vi "mappingProgramPublish.vi"() -> ()   [LabVIEW 2023]
uses:
  <vilib>/Math Plots/3D Math Plots/3D Comet/3D Comet XCtrl/3D Comet.xctl
  Program Files/National Instruments/LabVIEW 2023/examples/Instrument IO/Serial/support/Serial - Settings.ctl
  <vilib>/Instr/_visa.llb/VISA Configure Serial Port (Instr).vi
  <vilib>/Utility/file.llb/Read Delimited Spreadsheet (DBL).vi
  <vilib>/Math Plots/3D Math Plots/3D Comet/3D Comet Datatype/Public/Plot Helper (Matrices).vi
  Program Files/National Instruments/LabVIEW 2023/instr.lib/Marlin Instrument Driver/Marlin Instrument Driver.lvlib
  <vilib>/Math Plots/3D Math Plots/3D Comet/3D Comet Datatype/3D Comet Datatype.lvclass
panel:
  in  "Plot Path Button":bool
  out "MAPPING PATH VISUALIZER (mm)":refnum<class "3D Plot Datatype.lvclass">[](xcontrol)
  in  "Data Save Location":path
  in  "Close Probe\nClose 2":bool
  in  "Probe COM port":refnum<visa-resource-name>
  in  "Path":path caption="Pathing File Location"
  in  "Run Scan":bool
  in  "Custom Command":string
  out "Z":string
  out "Y":string
  out "X":string
  in  "Exit Scan\nClose":bool caption="Close\nClose"
  out "Initialized":bool
  in  "Initialize":bool
  in  "COM port":refnum<visa-resource-name> caption="Printer Chassis COM port"
  in  "Speed":u32=1000 caption="mm/min"
  in  "Distance":dbl=2.0 caption="mm"
  in  "Home all":bool caption="ALL"
  in  "Home Z":bool
  in  "Z-":bool
  in  "Z+":bool
  in  "Home XY":bool
  in  "XY-":bool
  in  "X-":bool
  in  "XY+":bool
  in  "X-Y+":bool
  in  "Y-":bool
  in  "X+Y-":bool
  in  "X+":bool
  in  "Y+":bool
  # "ENSURE DATA SAVING LOCATION, PATHING FILE LOCATION, AND COM PORTS ARE SELECTED, \nAND PRINTER CHASSIS IS INITALIZED BEFORE ATTEMPTING TO RUN SCAN."
  # "CAUTION: Z-AXIS MOVEMENT MAY CRASH SENSOR INTO PRINT BED."
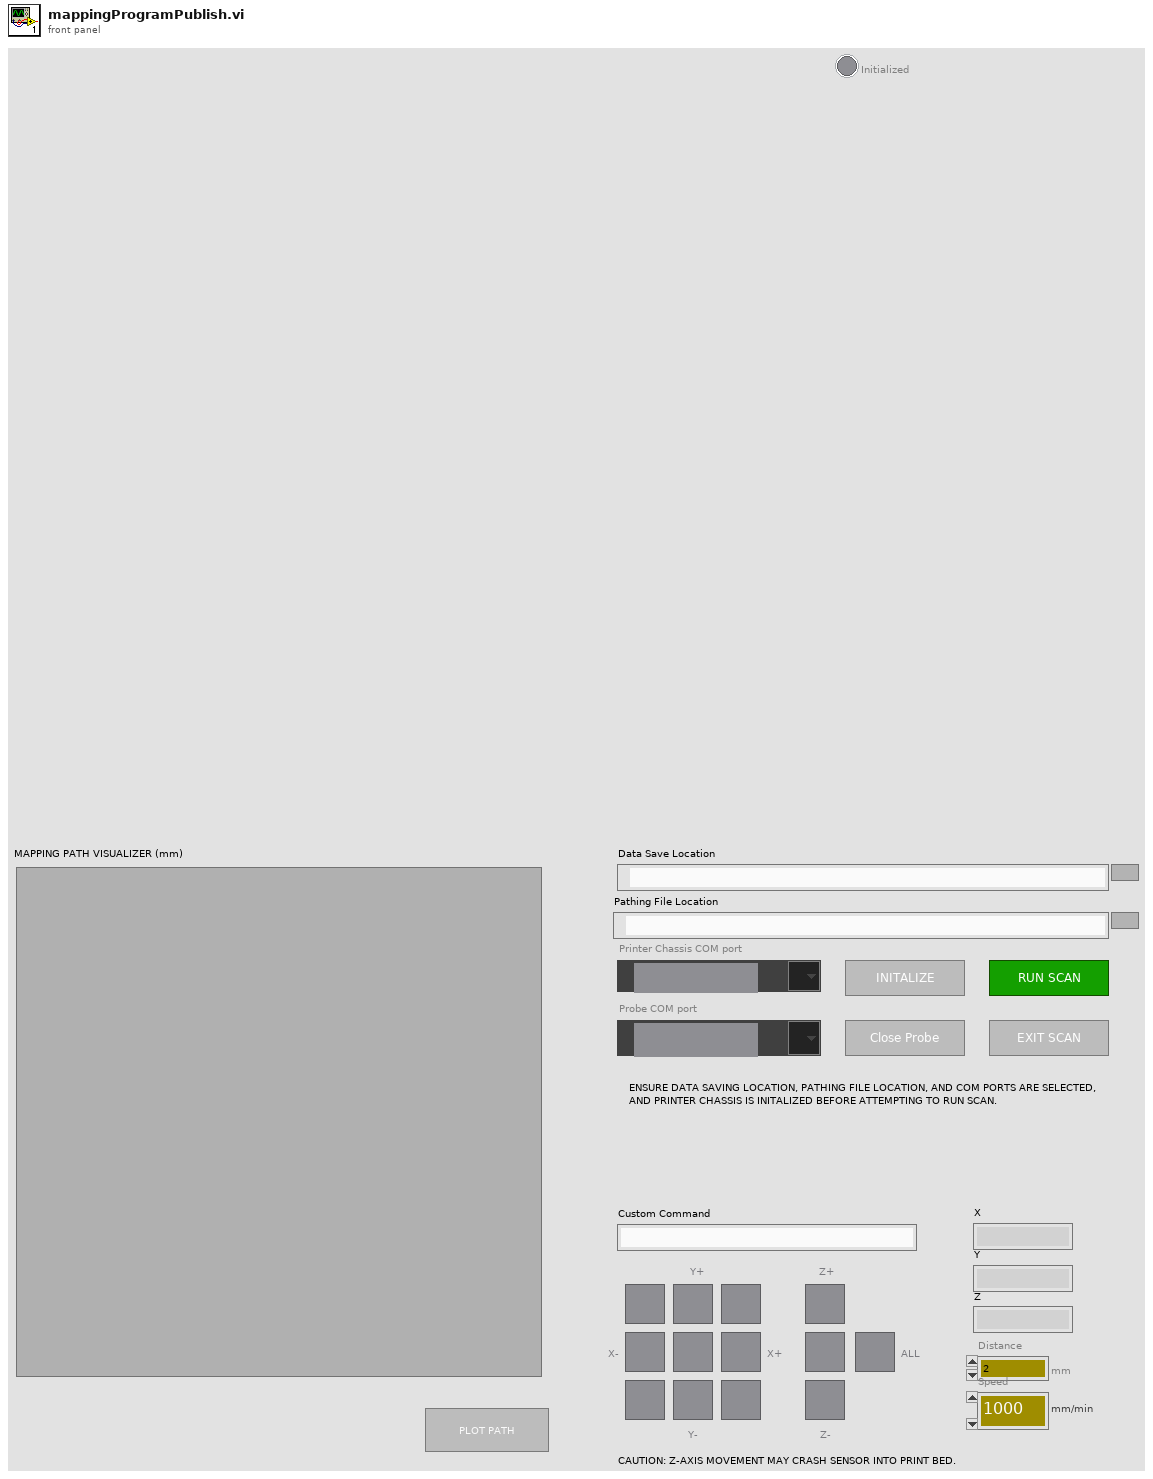
[diagram p1: front panel]
types:
  T1 = enum16{"open", "replace", "create", "open or create", "replace or create", "replace or create with confirmation"}
  T2 = typedef "Serial - Settings.ctl" = cluster{"baud rate":u32, "data bits":u16, "parity":enum16{"None", "Odd", "Even", "Mark", "Space"}, "stop bits":u16, "flow control":u16}
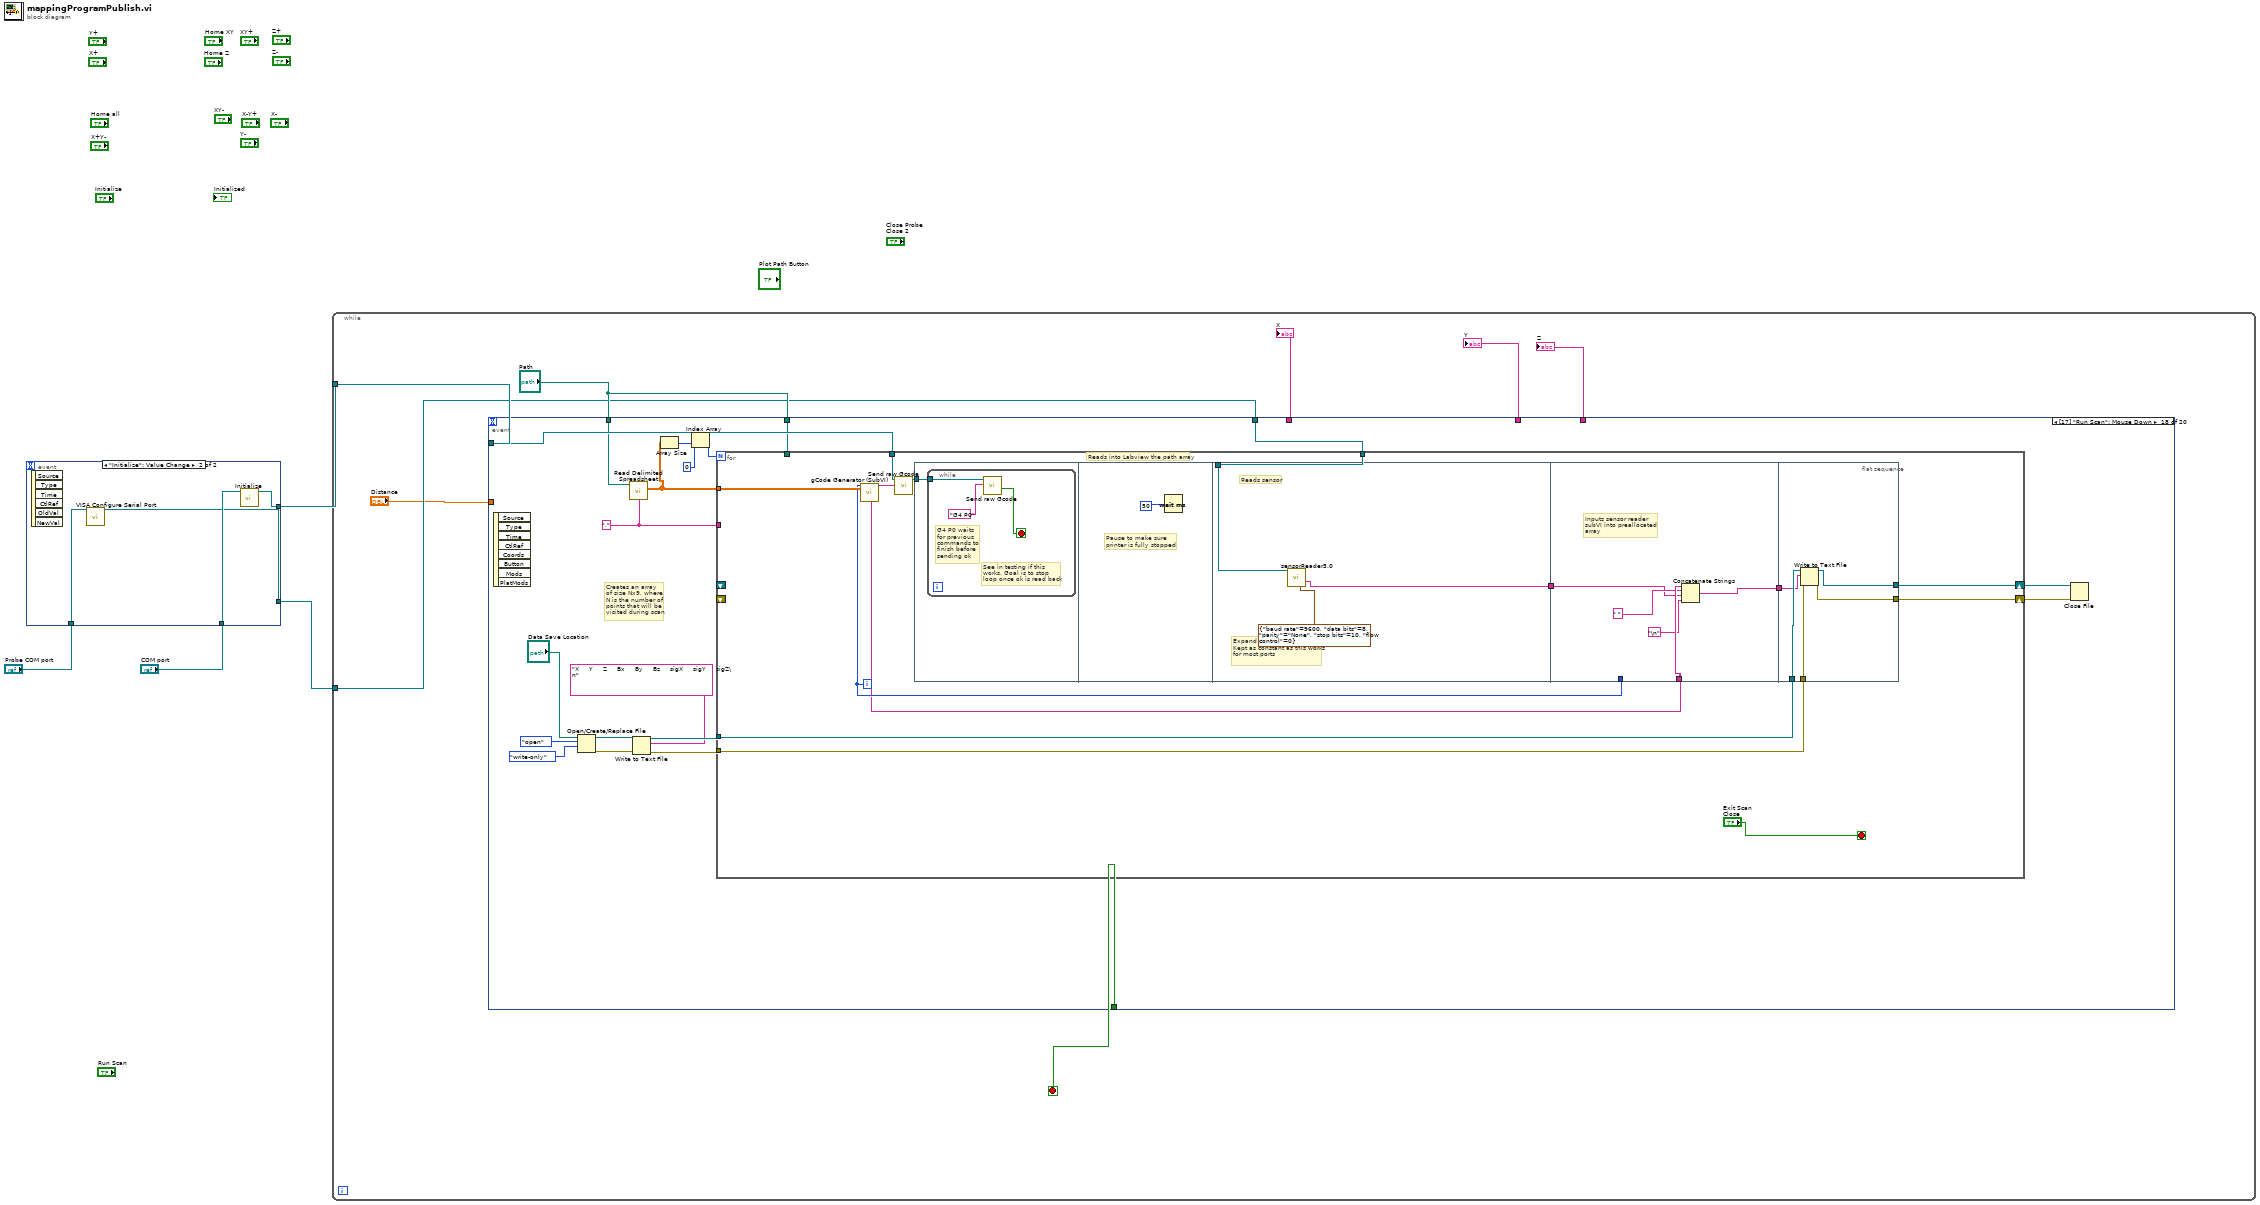
[diagram p0: block diagram]
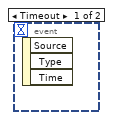
[diagram p2: hidden frame]
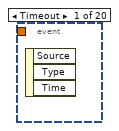
[diagram p3: hidden frame]
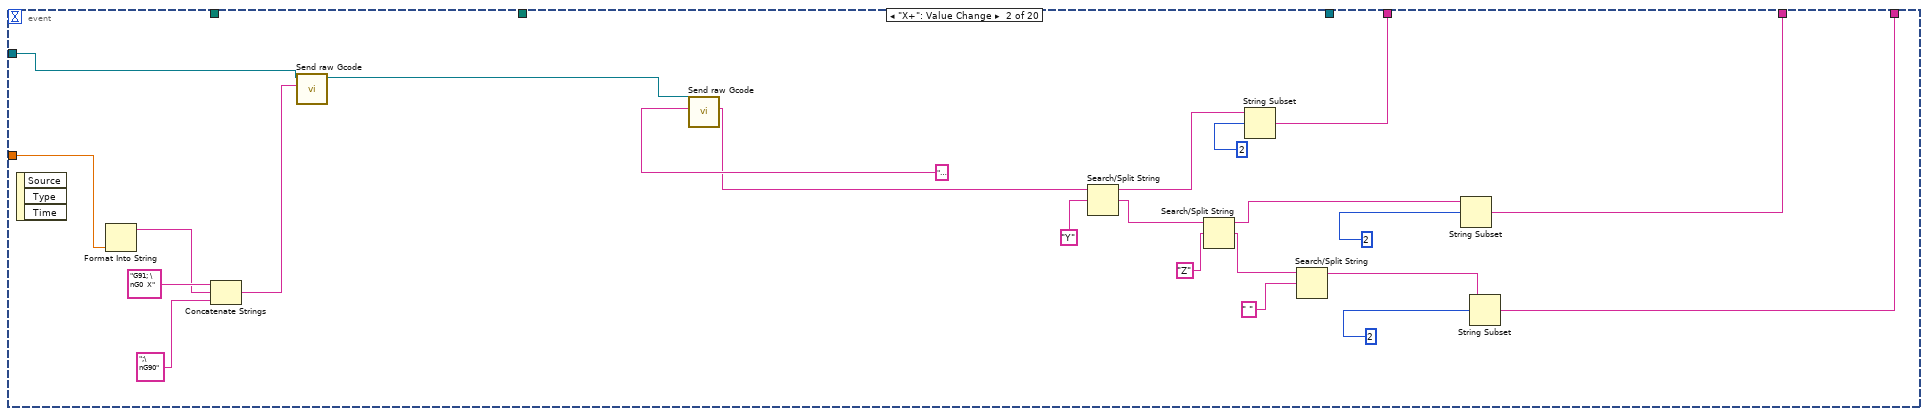
[diagram p4: hidden frame]
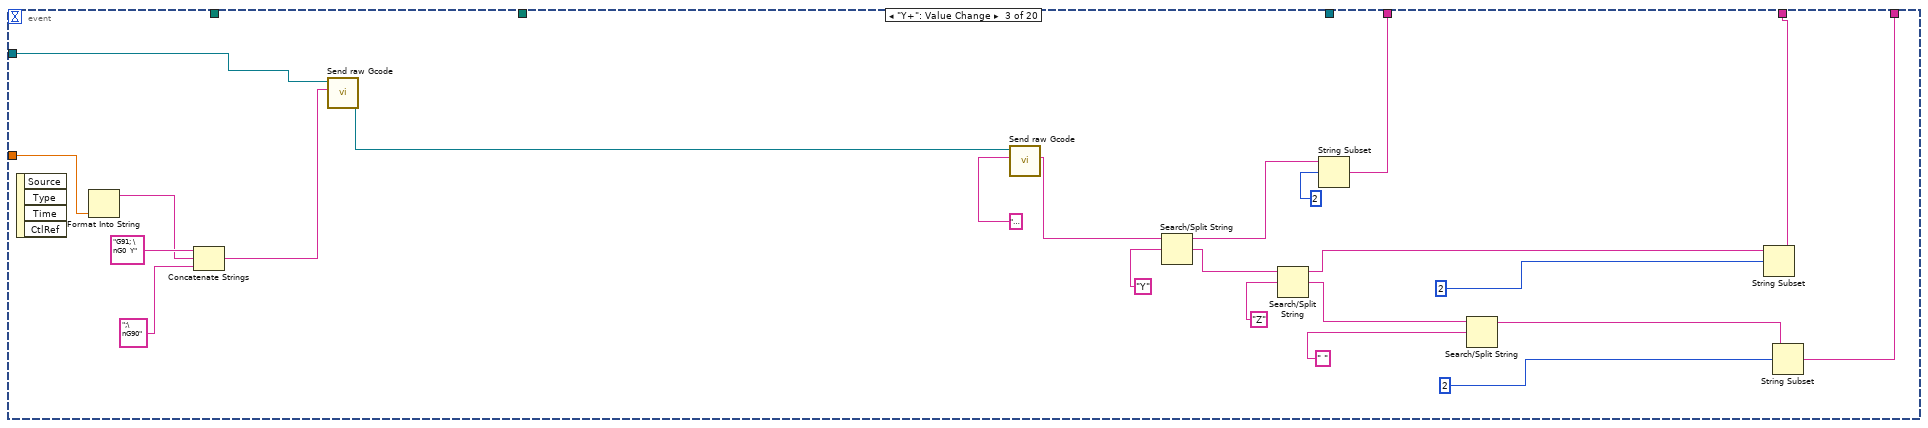
[diagram p5: hidden frame]
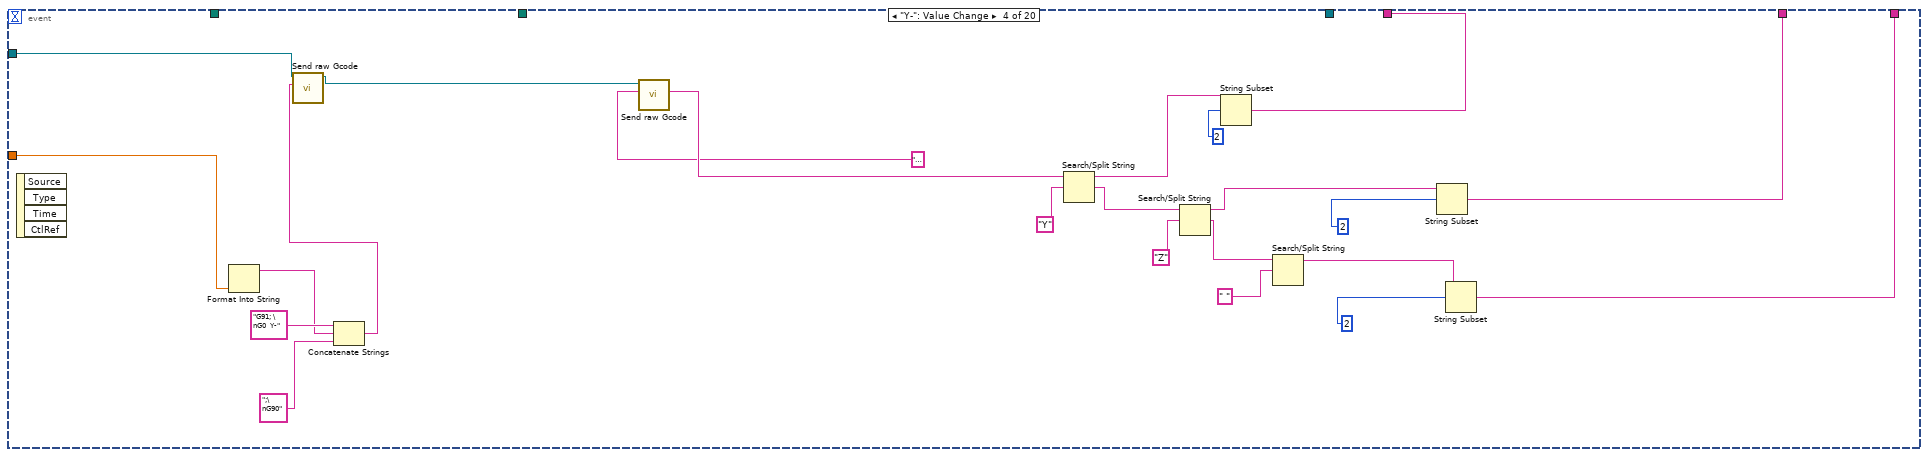
[diagram p6: hidden frame]
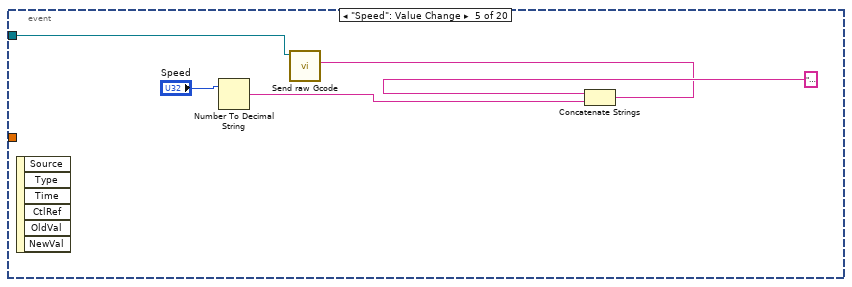
[diagram p7: hidden frame]
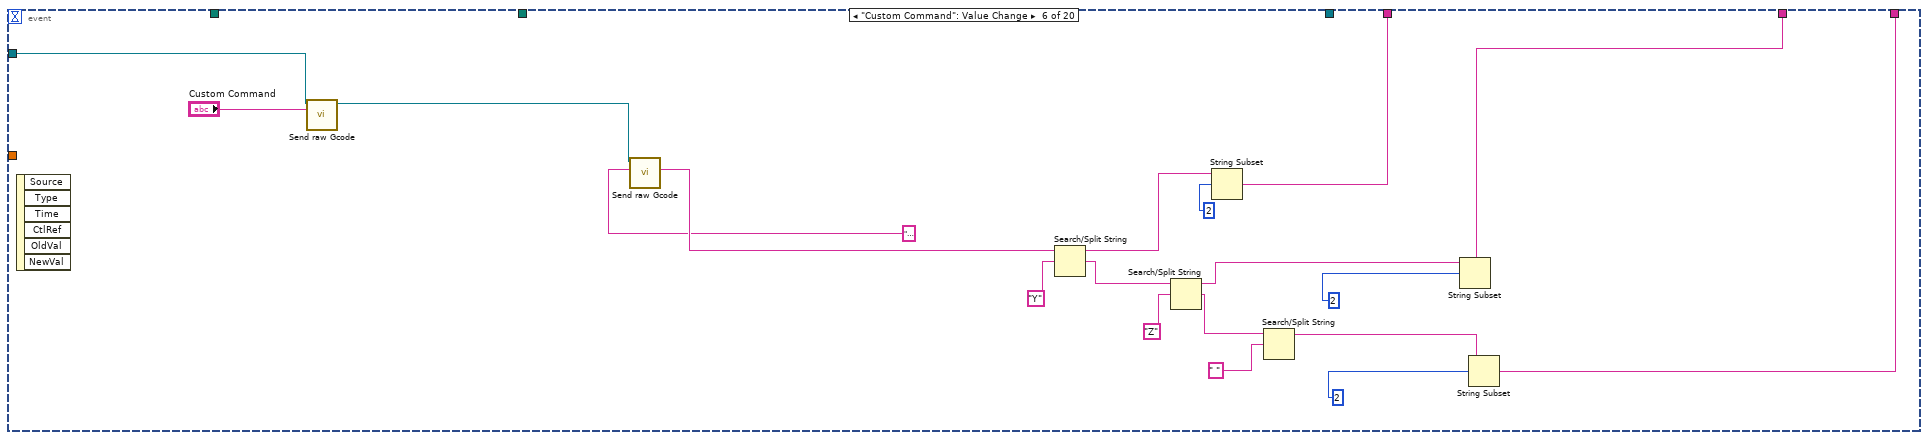
[diagram p8: hidden frame]
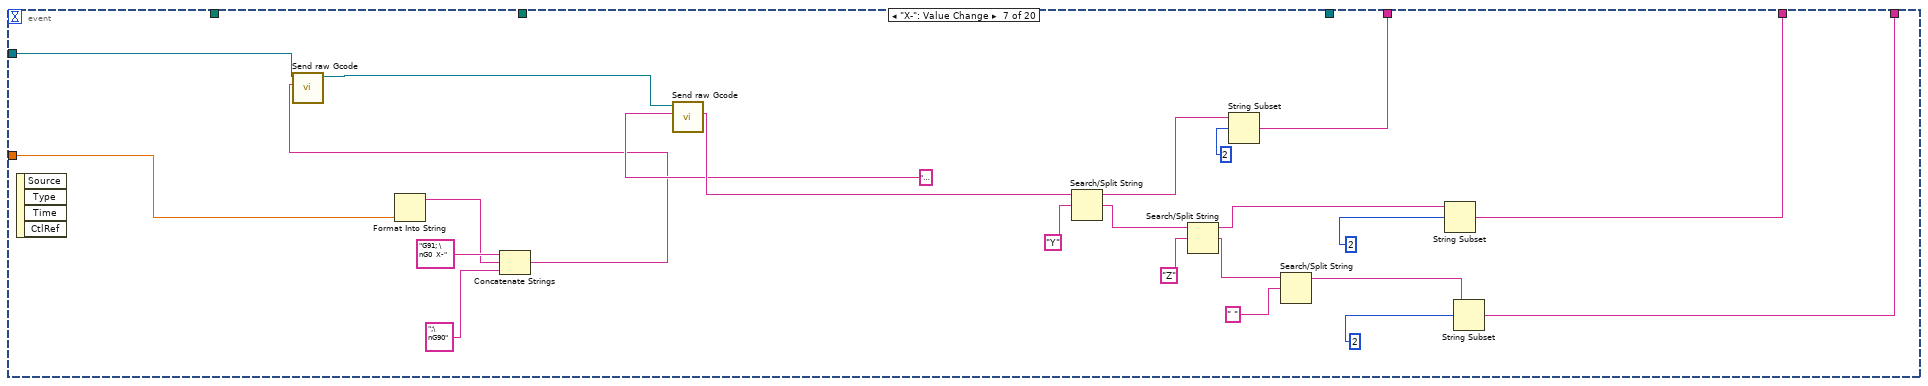
[diagram p9: hidden frame]
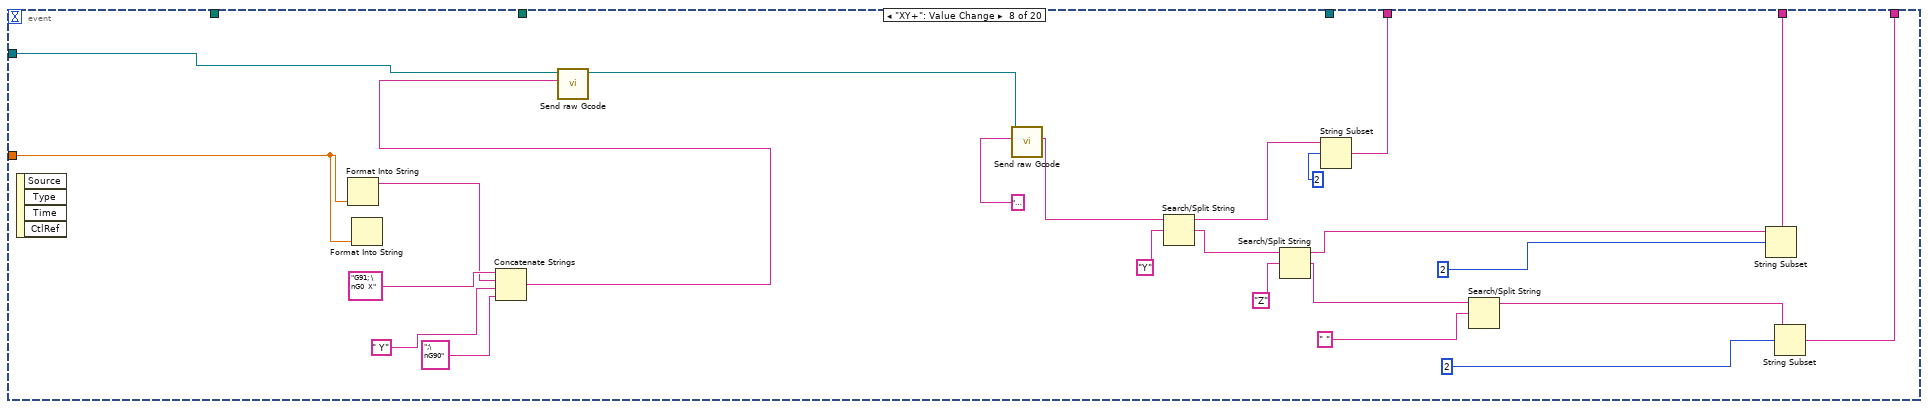
[diagram p10: hidden frame]
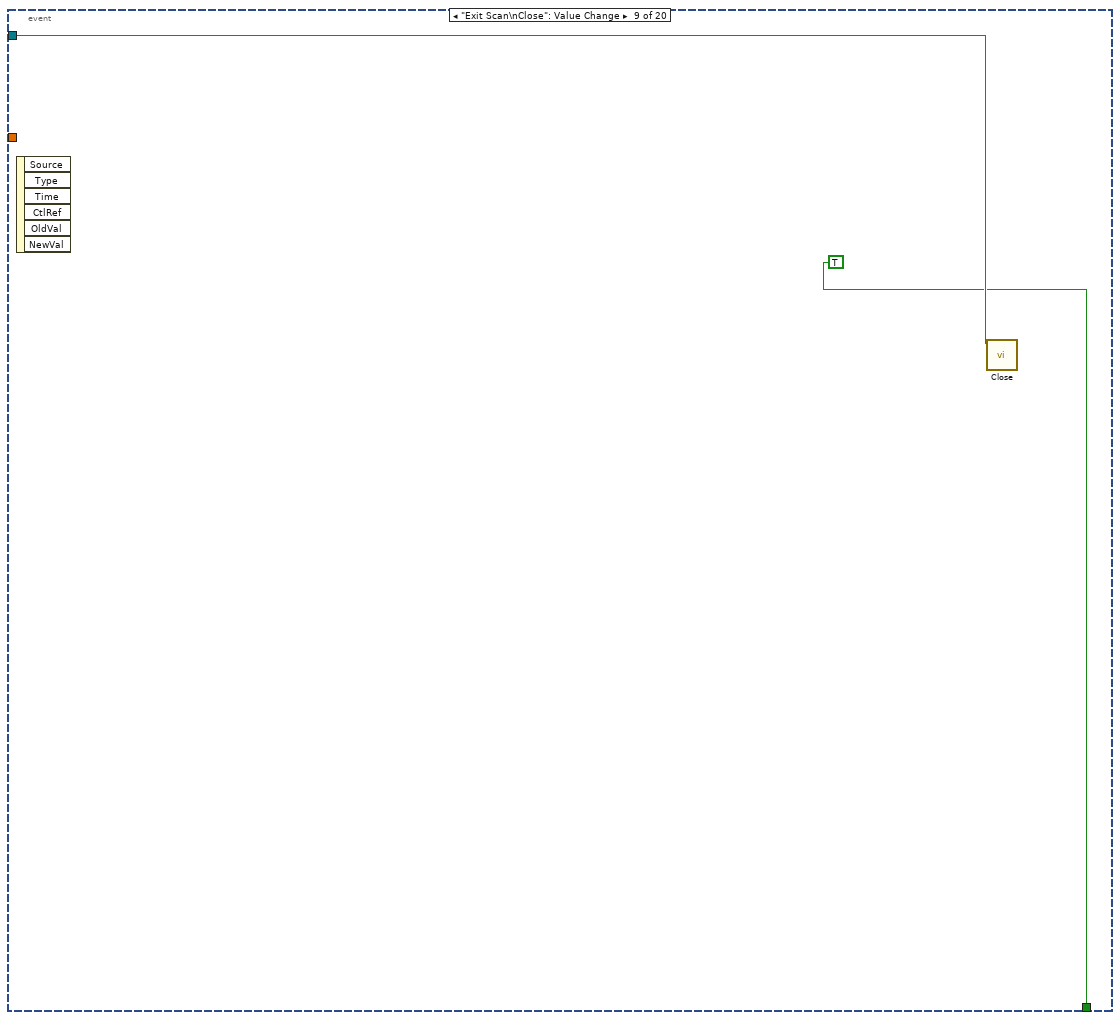
[diagram p11: hidden frame]
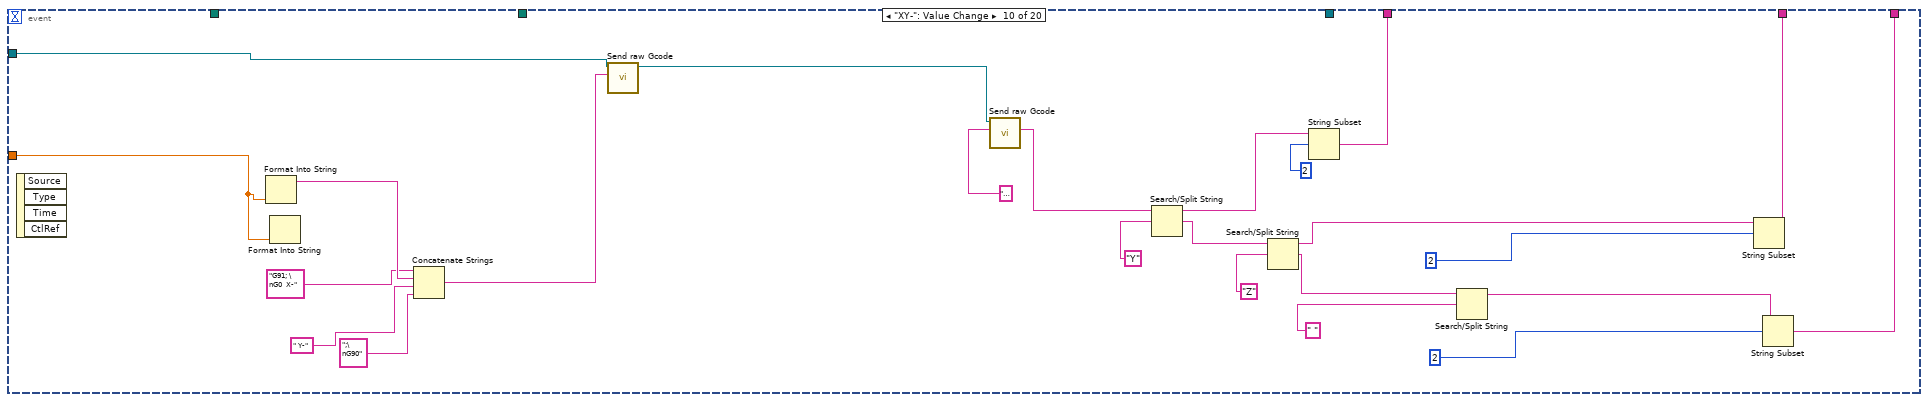
[diagram p12: hidden frame]
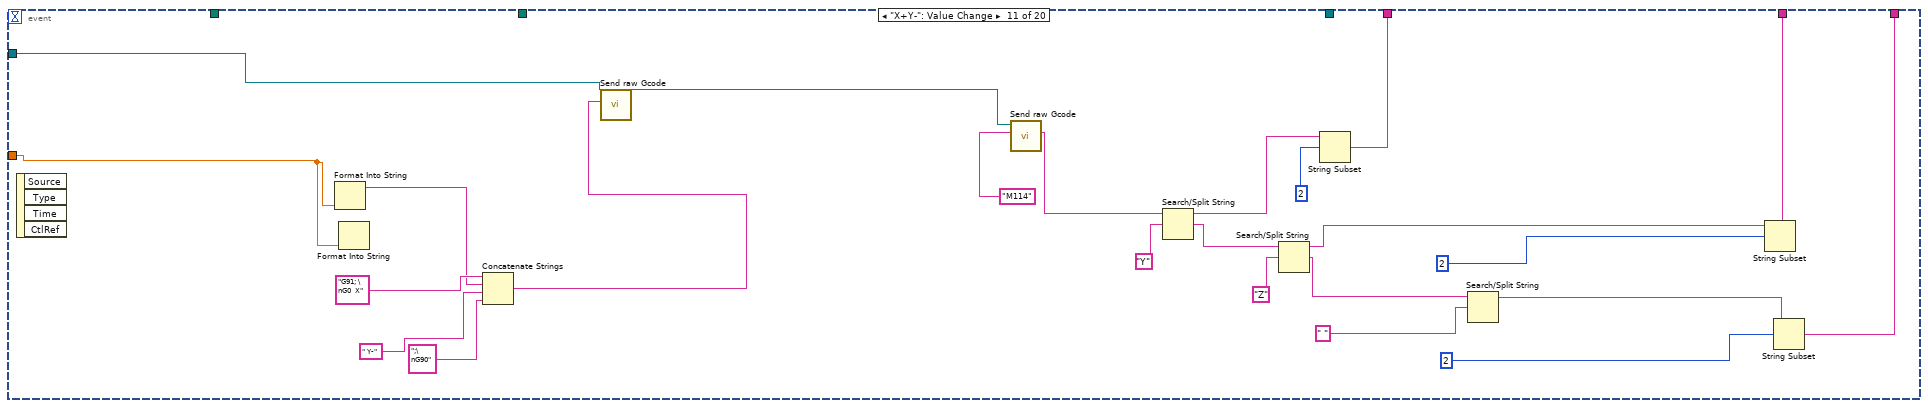
[diagram p13: hidden frame]
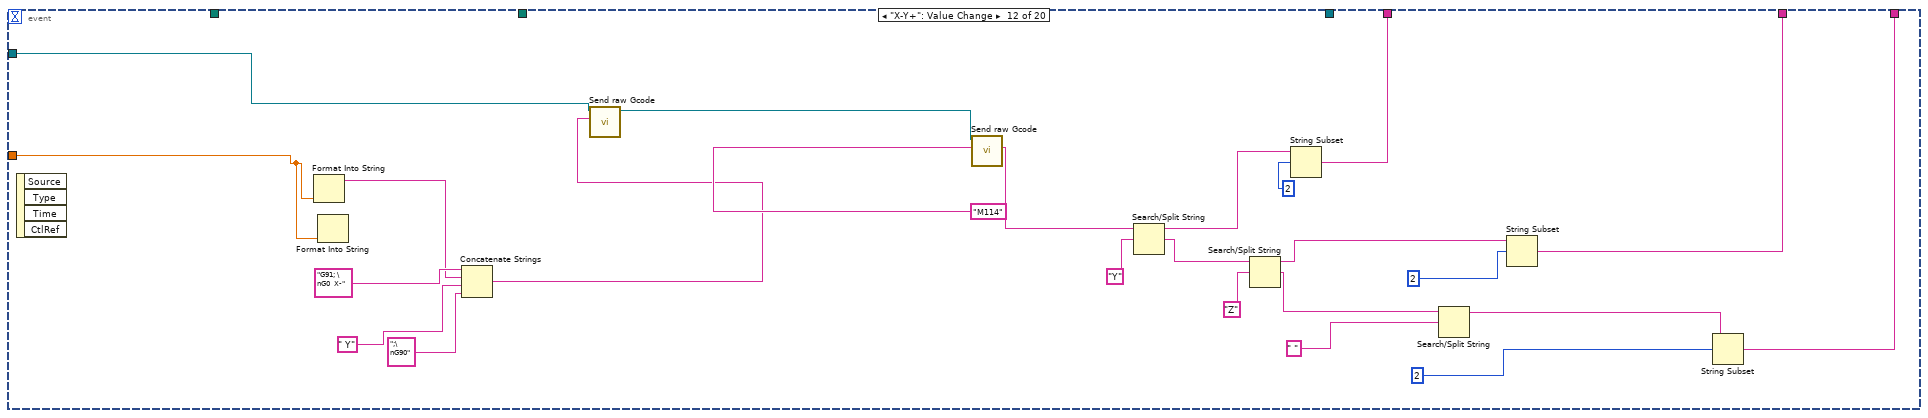
[diagram p14: hidden frame]
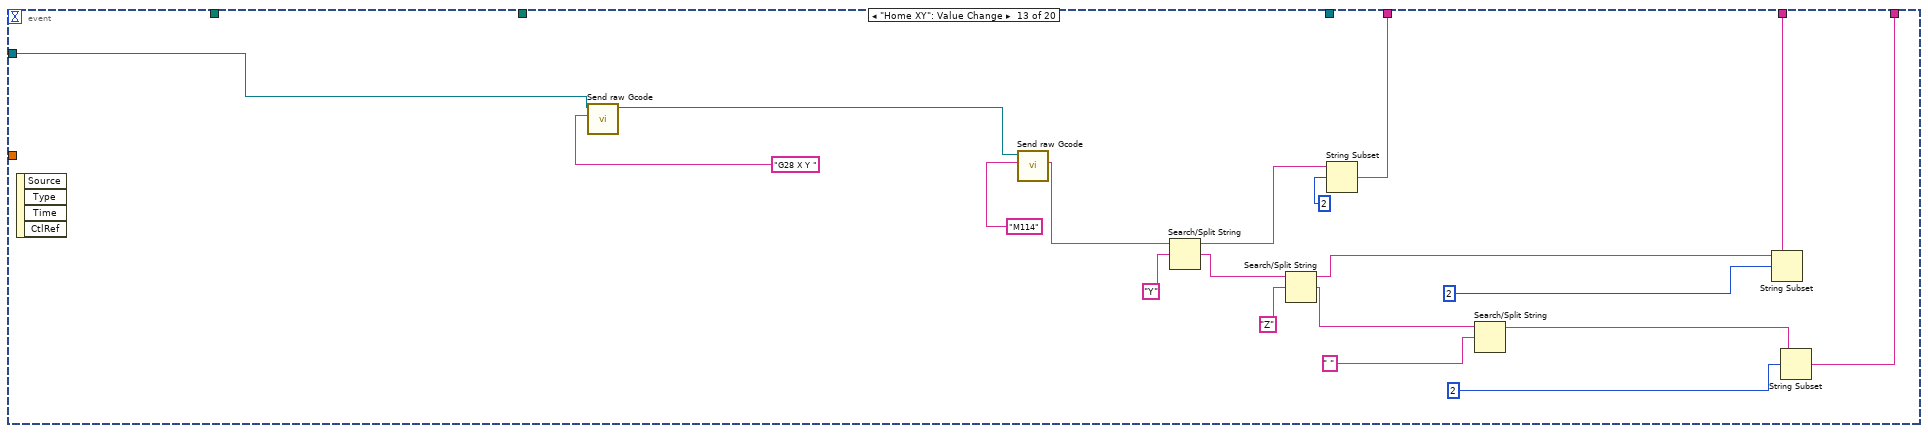
[diagram p15: hidden frame]
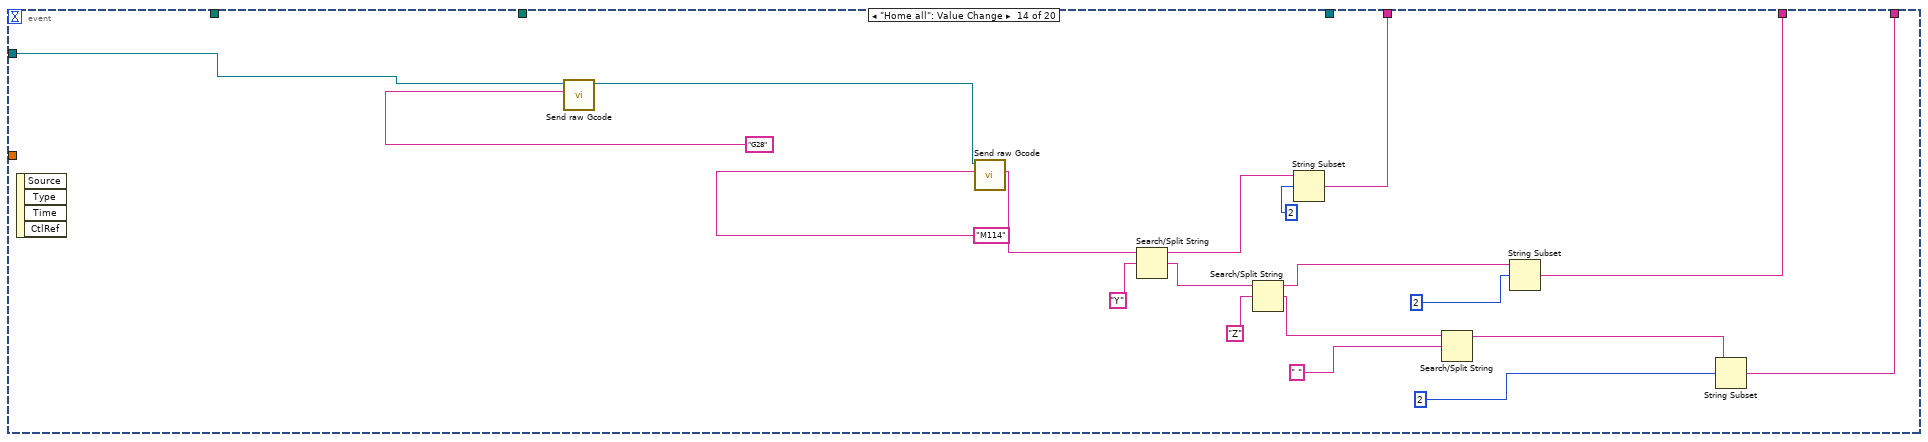
[diagram p16: hidden frame]
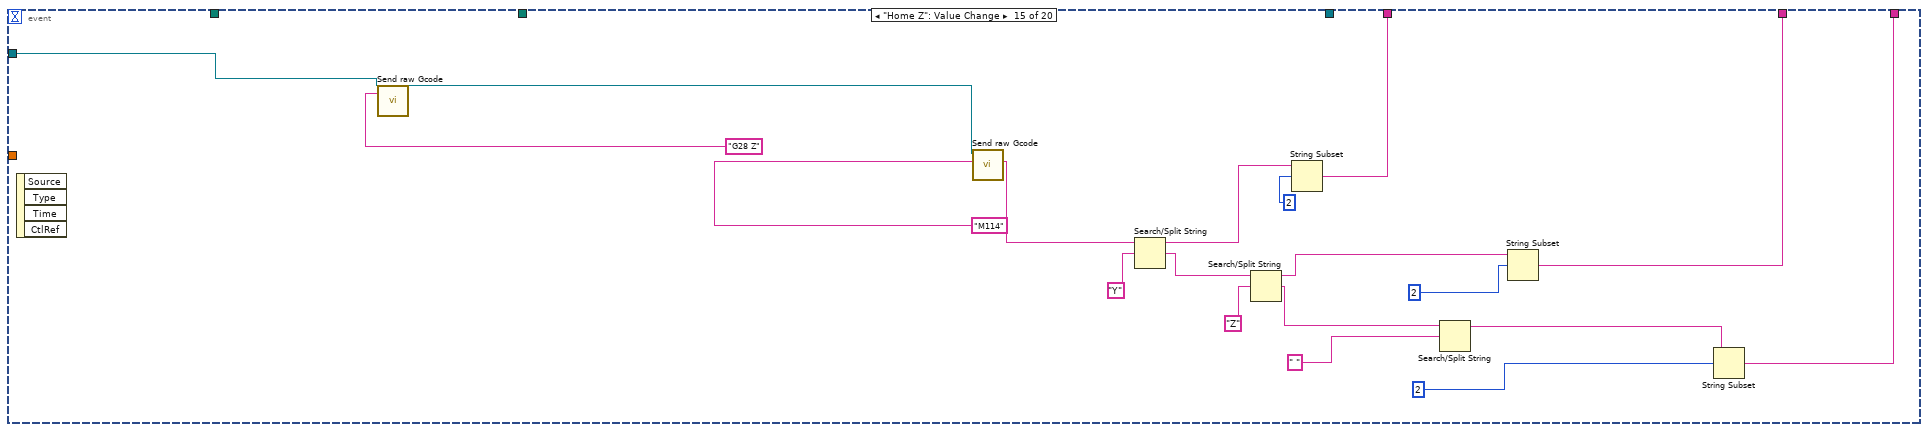
[diagram p17: hidden frame]
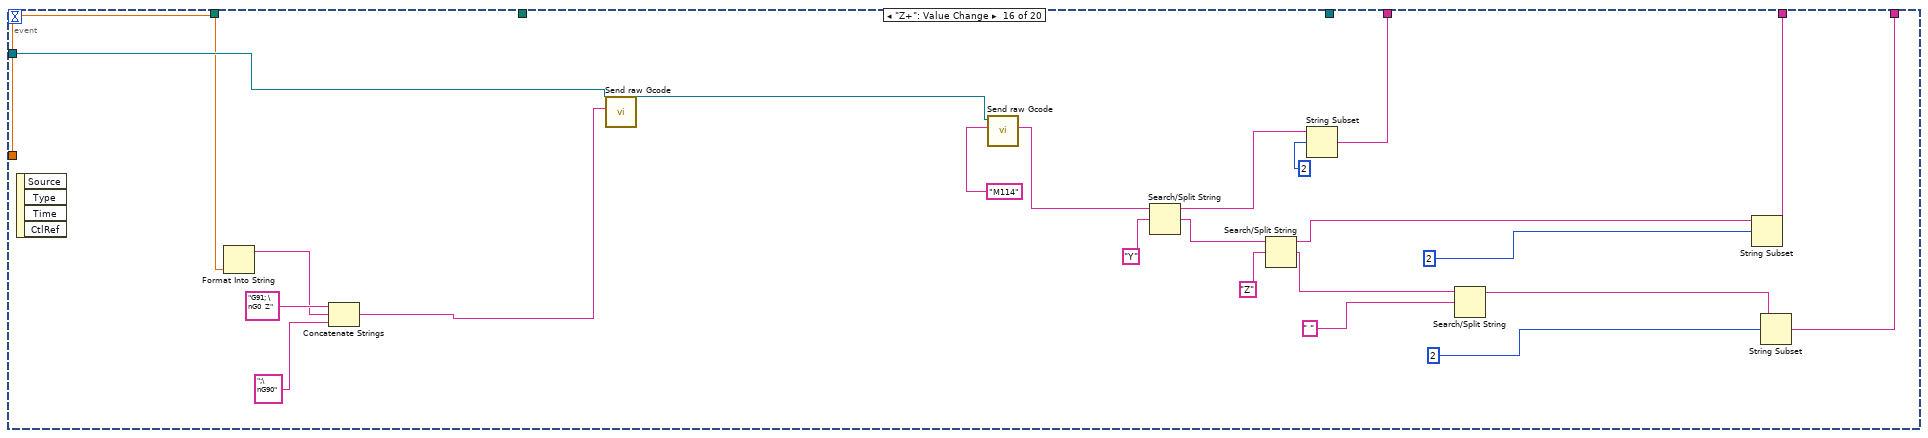
[diagram p18: hidden frame]
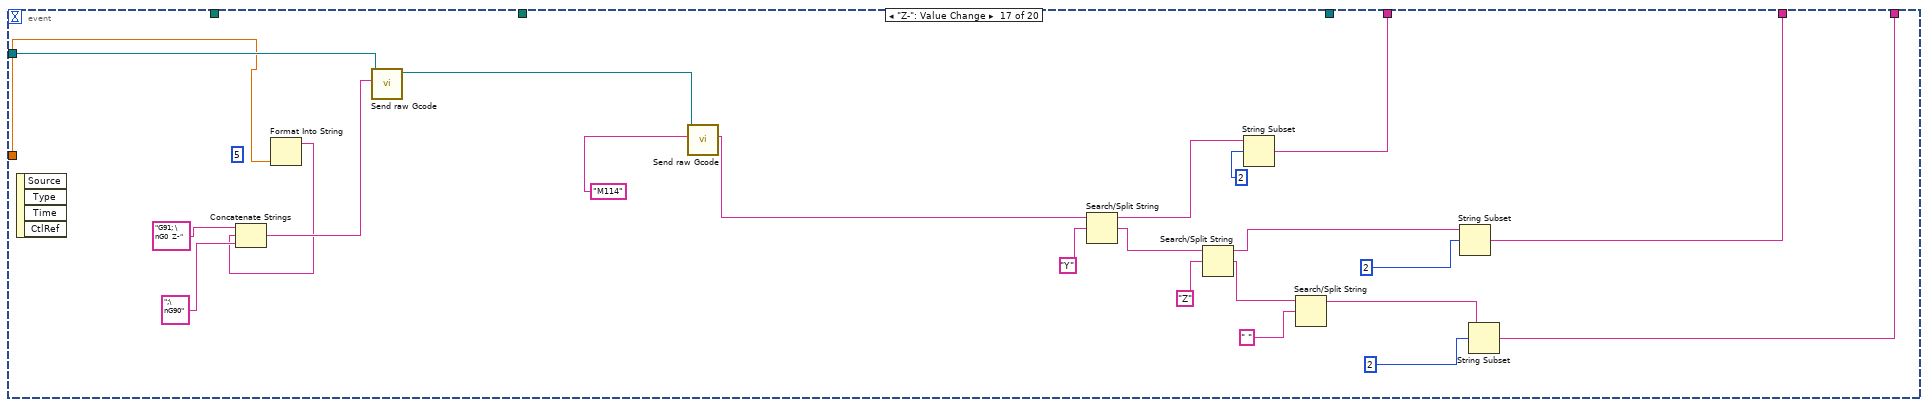
[diagram p19: hidden frame]
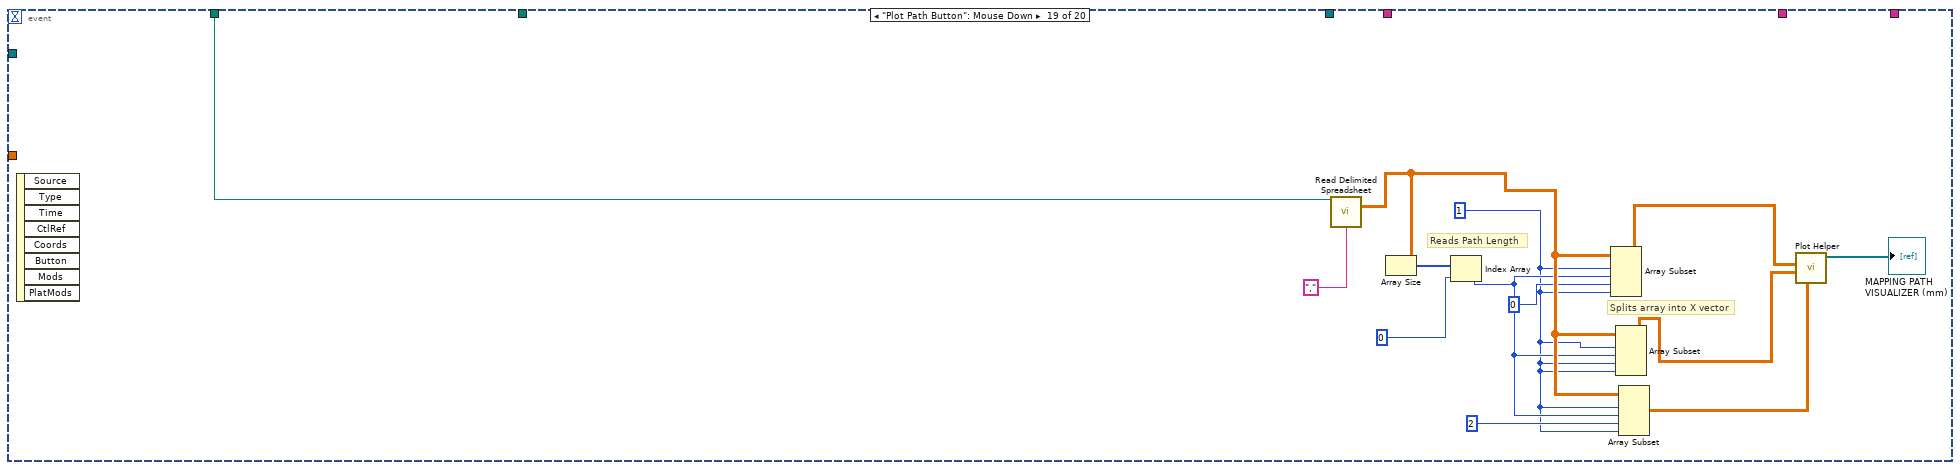
[diagram p20: hidden frame]
diagram:
  n1 = event shown="[1] \"Initialize\": Value Change" {
    selector: _ -> [_ _]
    dyn-events: _ -> [_ _]
    timeout: _ -> [_ _]
    tunnel: [_ w8] -> w3
    tunnel: "COM port" -> [_ w7]
    tunnel: "Probe COM port" -> [_ w6]
    tunnel: [_ w5] -> w1
    event Timeout {
      n2 = event-data() -> ()  [unwired: 1 in, 3 out]
    }
    event "Initialize": Value Change {
      n3 = event-data() -> ()  [unwired: 1 in, 6 out]
      n4 = call-poly "VISA Configure Serial Port"("VISA resource name"=w6) -> ("VISA resource name out"=w5:refnum<visa-resource-name>)  [unwired: 13 in, 1 out]
      n5 = call "Initialize.vi"("VISA resource name"=w7) -> ("VISA resource name out"=w8:refnum<visa-resource-name>)  [unwired: 9 in, 1 out]
    }
  }
  n6 = while {
    tunnel: w3 -> [w16]
    tunnel: w1 -> [w10]
    stop <- w15 stop-if-true
    n7 = event shown="[17] \"Run Scan\": Mouse Down" {
      selector: _ -> [_ _ _ _ _ _ _ _ _ _ _ _ _ _ _ _ _ _ _ _]
      dyn-events: _ -> [_ _ _ _ _ _ _ _ _ _ _ _ _ _ _ _ _ _ _ _]
      timeout: _ -> [_ _ _ _ _ _ _ _ _ _ _ _ _ _ _ _ _ _ _ _]
      tunnel: w16 -> [_ w38 w62 w85 w88 w109 w132 w156 w158 w182 w206 w230 w248 w267 w286 w310 w333 w351 _ _]
      tunnel: [_ _ _ _ _ _ _ _ TRUE _ _ _ _ _ _ _ _ _ _ _] -> w15
      tunnel: [_ w26 w47 w70 _ w94 w117 w141 _ w167 w191 w215 w233 w252 w271 w295 w318 _ _ _] -> w14
      tunnel: [_ w25 w46 w69 _ w93 w116 w140 _ w166 w190 w214 w232 w251 w270 w294 w317 _ _ _] -> w13
      tunnel: [_ w24 w45 w68 _ w92 w115 w139 _ w165 w189 w213 w231 w250 w269 w293 w316 _ _ _] -> w12
      tunnel: w10 -> [_ _ _ _ _ _ _ _ _ _ _ _ _ _ _ _ _ w348 _ w398]
      tunnel: "Path" -> [_ _ _ _ _ _ _ _ _ _ _ _ _ _ _ _ _ w346 w385 _]
      tunnel: "Path" -> [_ _ _ _ _ _ _ _ _ _ _ _ _ _ _ _ _ w345 _ _]
      tunnel: "Distance" -> [_ w17 w40 w63 _ _ w110 w137 _ w160 w184 w208 _ _ _ w289 w312 _ _ _]
      event Timeout {
        n8 = event-data() -> ()  [unwired: 1 in, 3 out]
      }
      event "X+": Value Change {
        n9 = event-data() -> ()  [unwired: 1 in, 3 out]
        n10 = Format Into String(w17) -> (resulting string=w19:string)  [unwired: 3 in, 1 out]
        n11 = Concatenate Strings("G91; \nG0  X", w19, ";\nG90") -> (w18:string)
        n12 = call "Send raw Gcode.vi"("Gcode"=w18, "VISA resource name"=w38) -> ("VISA resource name out"=w22:refnum<visa-resource-name>)  [unwired: 6 in, 3 out]
        n13 = call "Send raw Gcode.vi"("Gcode"="M114", "VISA resource name"=w22) -> ("read buffer"=w23:string)  [unwired: 6 in, 3 out]
        n14 = Search/Split String(string=w23, search string/char (-)="Y") -> (substring before match=w28:string, match + rest of string=w27:string)  [unwired: 1 in, 1 out]
        n15 = Search/Split String(string=w27, search string/char (-)="Z") -> (substring before match=w30:string, match + rest of string=w31:string)  [unwired: 1 in, 1 out]
        n16 = String Subset(string=w28, offset (0)=2) -> (substring=w26:string)  [unwired: 1 in]
        n17 = Search/Split String(string=w31, search string/char (-)=" ") -> (substring before match=w29:string)  [unwired: 1 in, 2 out]
        n18 = String Subset(string=w30, offset (0)=2) -> (substring=w25:string)  [unwired: 1 in]
        n19 = String Subset(string=w29, offset (0)=2) -> (substring=w24:string)  [unwired: 1 in]
      }
      event "Y+": Value Change {
        n20 = event-data() -> ()  [unwired: 1 in, 4 out]
        n21 = Format Into String(w40) -> (resulting string=w42:string)  [unwired: 3 in, 1 out]
        n22 = Concatenate Strings("G91; \nG0  Y", w42, ";\nG90") -> (w41:string)
        n23 = call "Send raw Gcode.vi"("Gcode"=w41, "VISA resource name"=w62) -> ("VISA resource name out"=w48:refnum<visa-resource-name>)  [unwired: 6 in, 3 out]
        n24 = call "Send raw Gcode.vi"("Gcode"="M114", "VISA resource name"=w48) -> ("read buffer"=w61:string)  [unwired: 6 in, 3 out]
        n25 = Search/Split String(string=w61, search string/char (-)="Y") -> (substring before match=w59:string, match + rest of string=w60:string)  [unwired: 1 in, 1 out]
        n26 = Search/Split String(string=w60, search string/char (-)="Z") -> (substring before match=w57:string, match + rest of string=w56:string)  [unwired: 1 in, 1 out]
        n27 = String Subset(string=w59, offset (0)=2) -> (substring=w47:string)  [unwired: 1 in]
        n28 = Search/Split String(string=w56, search string/char (-)=" ") -> (substring before match=w58:string)  [unwired: 1 in, 2 out]
        n29 = String Subset(string=w57, offset (0)=2) -> (substring=w46:string)  [unwired: 1 in]
        n30 = String Subset(string=w58, offset (0)=2) -> (substring=w45:string)  [unwired: 1 in]
      }
      event "Y-": Value Change {
        n31 = event-data() -> ()  [unwired: 1 in, 4 out]
        n32 = Format Into String(w63) -> (resulting string=w65:string)  [unwired: 3 in, 1 out]
        n33 = Concatenate Strings("G91; \nG0  Y-", w65, ";\nG90") -> (w64:string)
        n34 = call "Send raw Gcode.vi"("Gcode"=w64, "VISA resource name"=w85) -> ("VISA resource name out"=w71:refnum<visa-resource-name>)  [unwired: 6 in, 3 out]
        n35 = call "Send raw Gcode.vi"("Gcode"="M114", "VISA resource name"=w71) -> ("read buffer"=w79:string)  [unwired: 6 in, 3 out]
        n36 = Search/Split String(string=w79, search string/char (-)="Y") -> (substring before match=w81:string, match + rest of string=w80:string)  [unwired: 1 in, 1 out]
        n37 = Search/Split String(string=w80, search string/char (-)="Z") -> (substring before match=w83:string, match + rest of string=w84:string)  [unwired: 1 in, 1 out]
        n38 = String Subset(string=w81, offset (0)=2) -> (substring=w70:string)  [unwired: 1 in]
        n39 = Search/Split String(string=w84, search string/char (-)=" ") -> (substring before match=w82:string)  [unwired: 1 in, 2 out]
        n40 = String Subset(string=w83, offset (0)=2) -> (substring=w69:string)  [unwired: 1 in]
        n41 = String Subset(string=w82, offset (0)=2) -> (substring=w68:string)  [unwired: 1 in]
      }
      event "Speed": Value Change {
        n42 = event-data() -> ()  [unwired: 1 in, 6 out]
        n43 = Number To Decimal String(number="Speed") -> (decimal integer string=w89:string)  [unwired: 1 in]
        n44 = Concatenate Strings("G0 F", w89) -> (w86:string)
        n45 = call "Send raw Gcode.vi"("Gcode"=w86, "VISA resource name"=w88) -> ()  [unwired: 6 in, 4 out]
      }
      event "Custom Command": Value Change {
        n46 = event-data() -> ()  [unwired: 1 in, 6 out]
        n47 = call "Send raw Gcode.vi"("Gcode"="Custom Command", "VISA resource name"=w109) -> ("VISA resource name out"=w91:refnum<visa-resource-name>)  [unwired: 6 in, 3 out]
        n48 = call "Send raw Gcode.vi"("Gcode"="M114", "VISA resource name"=w91) -> ("read buffer"=w102:string)  [unwired: 6 in, 3 out]
        n49 = Search/Split String(string=w102, search string/char (-)="Y") -> (substring before match=w104:string, match + rest of string=w103:string)  [unwired: 1 in, 1 out]
        n50 = Search/Split String(string=w103, search string/char (-)="Z") -> (substring before match=w106:string, match + rest of string=w107:string)  [unwired: 1 in, 1 out]
        n51 = String Subset(string=w104, offset (0)=2) -> (substring=w94:string)  [unwired: 1 in]
        n52 = Search/Split String(string=w107, search string/char (-)=" ") -> (substring before match=w105:string)  [unwired: 1 in, 2 out]
        n53 = String Subset(string=w106, offset (0)=2) -> (substring=w93:string)  [unwired: 1 in]
        n54 = String Subset(string=w105, offset (0)=2) -> (substring=w92:string)  [unwired: 1 in]
      }
      event "X-": Value Change {
        n55 = event-data() -> ()  [unwired: 1 in, 4 out]
        n56 = Format Into String(w110) -> (resulting string=w112:string)  [unwired: 3 in, 1 out]
        n57 = Concatenate Strings("G91; \nG0  X-", w112, ";\nG90") -> (w111:string)
        n58 = call "Send raw Gcode.vi"("Gcode"=w111, "VISA resource name"=w132) -> ("VISA resource name out"=w118:refnum<visa-resource-name>)  [unwired: 6 in, 3 out]
        n59 = call "Send raw Gcode.vi"("Gcode"="M114", "VISA resource name"=w118) -> ("read buffer"=w126:string)  [unwired: 6 in, 3 out]
        n60 = Search/Split String(string=w126, search string/char (-)="Y") -> (substring before match=w128:string, match + rest of string=w127:string)  [unwired: 1 in, 1 out]
        n61 = Search/Split String(string=w127, search string/char (-)="Z") -> (substring before match=w130:string, match + rest of string=w131:string)  [unwired: 1 in, 1 out]
        n62 = String Subset(string=w128, offset (0)=2) -> (substring=w117:string)  [unwired: 1 in]
        n63 = Search/Split String(string=w131, search string/char (-)=" ") -> (substring before match=w129:string)  [unwired: 1 in, 2 out]
        n64 = String Subset(string=w130, offset (0)=2) -> (substring=w116:string)  [unwired: 1 in]
        n65 = String Subset(string=w129, offset (0)=2) -> (substring=w115:string)  [unwired: 1 in]
      }
      event "XY+": Value Change {
        n66 = event-data() -> ()  [unwired: 1 in, 4 out]
        n67 = Format Into String(w137) -> (resulting string=w135:string)  [unwired: 3 in, 1 out]
        n68 = Format Into String(w137) -> ()  [unwired: 3 in, 2 out]
        n69 = Concatenate Strings("G91; \nG0  X", w135, " Y", ";\nG90") -> (w138:string)
        n70 = call "Send raw Gcode.vi"("Gcode"=w138, "VISA resource name"=w156) -> ("VISA resource name out"=w142:refnum<visa-resource-name>)  [unwired: 6 in, 3 out]
        n71 = call "Send raw Gcode.vi"("Gcode"="M114", "VISA resource name"=w142) -> ("read buffer"=w150:string)  [unwired: 6 in, 3 out]
        n72 = Search/Split String(string=w150, search string/char (-)="Y") -> (substring before match=w152:string, match + rest of string=w151:string)  [unwired: 1 in, 1 out]
        n73 = Search/Split String(string=w151, search string/char (-)="Z") -> (substring before match=w154:string, match + rest of string=w155:string)  [unwired: 1 in, 1 out]
        n74 = String Subset(string=w152, offset (0)=2) -> (substring=w141:string)  [unwired: 1 in]
        n75 = Search/Split String(string=w155, search string/char (-)=" ") -> (substring before match=w153:string)  [unwired: 1 in, 2 out]
        n76 = String Subset(string=w154, offset (0)=2) -> (substring=w140:string)  [unwired: 1 in]
        n77 = String Subset(string=w153, offset (0)=2) -> (substring=w139:string)  [unwired: 1 in]
      }
      event "Exit Scan\nClose": Value Change {
        n78 = event-data() -> ()  [unwired: 1 in, 6 out]
        n79 = call "Close.vi"("VISA resource name"=w158) -> ()  [unwired: 10 in, 1 out]
      }
      event "XY-": Value Change {
        n80 = event-data() -> ()  [unwired: 1 in, 4 out]
        n81 = Format Into String(w160) -> (resulting string=w164:string)  [unwired: 3 in, 1 out]
        n82 = Format Into String(w160) -> ()  [unwired: 3 in, 2 out]
        n83 = Concatenate Strings("G91; \nG0  X-", w164, " Y-", ";\nG90") -> (w159:string)
        n84 = call "Send raw Gcode.vi"("Gcode"=w159, "VISA resource name"=w182) -> ("VISA resource name out"=w168:refnum<visa-resource-name>)  [unwired: 6 in, 3 out]
        n85 = call "Send raw Gcode.vi"("Gcode"="M114", "VISA resource name"=w168) -> ("read buffer"=w181:string)  [unwired: 6 in, 3 out]
        n86 = Search/Split String(string=w181, search string/char (-)="Y") -> (substring before match=w179:string, match + rest of string=w180:string)  [unwired: 1 in, 1 out]
        n87 = Search/Split String(string=w180, search string/char (-)="Z") -> (substring before match=w177:string, match + rest of string=w176:string)  [unwired: 1 in, 1 out]
        n88 = String Subset(string=w179, offset (0)=2) -> (substring=w167:string)  [unwired: 1 in]
        n89 = Search/Split String(string=w176, search string/char (-)=" ") -> (substring before match=w178:string)  [unwired: 1 in, 2 out]
        n90 = String Subset(string=w177, offset (0)=2) -> (substring=w166:string)  [unwired: 1 in]
        n91 = String Subset(string=w178, offset (0)=2) -> (substring=w165:string)  [unwired: 1 in]
      }
      event "X+Y-": Value Change {
        n92 = event-data() -> ()  [unwired: 1 in, 4 out]
        n93 = Format Into String(w184) -> (resulting string=w187:string)  [unwired: 3 in, 1 out]
        n94 = Format Into String(w184) -> ()  [unwired: 3 in, 2 out]
        n95 = Concatenate Strings("G91; \nG0  X", w187, " Y-", ";\nG90") -> (w183:string)
        n96 = call "Send raw Gcode.vi"("Gcode"=w183, "VISA resource name"=w206) -> ("VISA resource name out"=w192:refnum<visa-resource-name>)  [unwired: 6 in, 3 out]
        n97 = call "Send raw Gcode.vi"("Gcode"="M114", "VISA resource name"=w192) -> ("read buffer"=w200:string)  [unwired: 6 in, 3 out]
        n98 = Search/Split String(string=w200, search string/char (-)="Y") -> (substring before match=w202:string, match + rest of string=w201:string)  [unwired: 1 in, 1 out]
        n99 = Search/Split String(string=w201, search string/char (-)="Z") -> (substring before match=w204:string, match + rest of string=w205:string)  [unwired: 1 in, 1 out]
        n100 = String Subset(string=w202, offset (0)=2) -> (substring=w191:string)  [unwired: 1 in]
        n101 = Search/Split String(string=w205, search string/char (-)=" ") -> (substring before match=w203:string)  [unwired: 1 in, 2 out]
        n102 = String Subset(string=w204, offset (0)=2) -> (substring=w190:string)  [unwired: 1 in]
        n103 = String Subset(string=w203, offset (0)=2) -> (substring=w189:string)  [unwired: 1 in]
      }
      event "X-Y+": Value Change {
        n104 = event-data() -> ()  [unwired: 1 in, 4 out]
        n105 = Format Into String(w208) -> (resulting string=w211:string)  [unwired: 3 in, 1 out]
        n106 = Format Into String(w208) -> ()  [unwired: 3 in, 2 out]
        n107 = Concatenate Strings("G91; \nG0  X-", w211, " Y", ";\nG90") -> (w207:string)
        n108 = call "Send raw Gcode.vi"("Gcode"=w207, "VISA resource name"=w230) -> ("VISA resource name out"=w216:refnum<visa-resource-name>)  [unwired: 6 in, 3 out]
        n109 = call "Send raw Gcode.vi"("Gcode"="M114", "VISA resource name"=w216) -> ("read buffer"=w224:string)  [unwired: 6 in, 3 out]
        n110 = Search/Split String(string=w224, search string/char (-)="Y") -> (substring before match=w226:string, match + rest of string=w225:string)  [unwired: 1 in, 1 out]
        n111 = Search/Split String(string=w225, search string/char (-)="Z") -> (substring before match=w228:string, match + rest of string=w229:string)  [unwired: 1 in, 1 out]
        n112 = String Subset(string=w226, offset (0)=2) -> (substring=w215:string)  [unwired: 1 in]
        n113 = Search/Split String(string=w229, search string/char (-)=" ") -> (substring before match=w227:string)  [unwired: 1 in, 2 out]
        n114 = String Subset(string=w228, offset (0)=2) -> (substring=w214:string)  [unwired: 1 in]
        n115 = String Subset(string=w227, offset (0)=2) -> (substring=w213:string)  [unwired: 1 in]
      }
      event "Home XY": Value Change {
        n116 = event-data() -> ()  [unwired: 1 in, 4 out]
        n117 = call "Send raw Gcode.vi"("Gcode"="G28 X Y ", "VISA resource name"=w248) -> ("VISA resource name out"=w234:refnum<visa-resource-name>)  [unwired: 6 in, 3 out]
        n118 = call "Send raw Gcode.vi"("Gcode"="M114", "VISA resource name"=w234) -> ("read buffer"=w242:string)  [unwired: 6 in, 3 out]
        n119 = Search/Split String(string=w242, search string/char (-)="Y") -> (substring before match=w244:string, match + rest of string=w243:string)  [unwired: 1 in, 1 out]
        n120 = Search/Split String(string=w243, search string/char (-)="Z") -> (substring before match=w246:string, match + rest of string=w247:string)  [unwired: 1 in, 1 out]
        n121 = String Subset(string=w244, offset (0)=2) -> (substring=w233:string)  [unwired: 1 in]
        n122 = Search/Split String(string=w247, search string/char (-)=" ") -> (substring before match=w245:string)  [unwired: 1 in, 2 out]
        n123 = String Subset(string=w246, offset (0)=2) -> (substring=w232:string)  [unwired: 1 in]
        n124 = String Subset(string=w245, offset (0)=2) -> (substring=w231:string)  [unwired: 1 in]
      }
      event "Home all": Value Change {
        n125 = event-data() -> ()  [unwired: 1 in, 4 out]
        n126 = call "Send raw Gcode.vi"("Gcode"="G28", "VISA resource name"=w267) -> ("VISA resource name out"=w253:refnum<visa-resource-name>)  [unwired: 6 in, 3 out]
        n127 = call "Send raw Gcode.vi"("Gcode"="M114", "VISA resource name"=w253) -> ("read buffer"=w261:string)  [unwired: 6 in, 3 out]
        n128 = Search/Split String(string=w261, search string/char (-)="Y") -> (substring before match=w263:string, match + rest of string=w262:string)  [unwired: 1 in, 1 out]
        n129 = Search/Split String(string=w262, search string/char (-)="Z") -> (substring before match=w265:string, match + rest of string=w266:string)  [unwired: 1 in, 1 out]
        n130 = String Subset(string=w263, offset (0)=2) -> (substring=w252:string)  [unwired: 1 in]
        n131 = Search/Split String(string=w266, search string/char (-)=" ") -> (substring before match=w264:string)  [unwired: 1 in, 2 out]
        n132 = String Subset(string=w265, offset (0)=2) -> (substring=w251:string)  [unwired: 1 in]
        n133 = String Subset(string=w264, offset (0)=2) -> (substring=w250:string)  [unwired: 1 in]
      }
      event "Home Z": Value Change {
        n134 = event-data() -> ()  [unwired: 1 in, 4 out]
        n135 = call "Send raw Gcode.vi"("Gcode"="G28 Z", "VISA resource name"=w286) -> ("VISA resource name out"=w272:refnum<visa-resource-name>)  [unwired: 6 in, 3 out]
        n136 = call "Send raw Gcode.vi"("Gcode"="M114", "VISA resource name"=w272) -> ("read buffer"=w280:string)  [unwired: 6 in, 3 out]
        n137 = Search/Split String(string=w280, search string/char (-)="Y") -> (substring before match=w282:string, match + rest of string=w281:string)  [unwired: 1 in, 1 out]
        n138 = Search/Split String(string=w281, search string/char (-)="Z") -> (substring before match=w284:string, match + rest of string=w285:string)  [unwired: 1 in, 1 out]
        n139 = String Subset(string=w282, offset (0)=2) -> (substring=w271:string)  [unwired: 1 in]
        n140 = Search/Split String(string=w285, search string/char (-)=" ") -> (substring before match=w283:string)  [unwired: 1 in, 2 out]
        n141 = String Subset(string=w284, offset (0)=2) -> (substring=w270:string)  [unwired: 1 in]
        n142 = String Subset(string=w283, offset (0)=2) -> (substring=w269:string)  [unwired: 1 in]
      }
      event "Z+": Value Change {
        n143 = event-data() -> ()  [unwired: 1 in, 4 out]
        n144 = Format Into String(w289) -> (resulting string=w288:string)  [unwired: 3 in, 1 out]
        n145 = Concatenate Strings("G91; \nG0  Z", w288, ";\nG90") -> (w290:string)
        n146 = call "Send raw Gcode.vi"("Gcode"=w290, "VISA resource name"=w310) -> ("VISA resource name out"=w296:refnum<visa-resource-name>)  [unwired: 6 in, 3 out]
        n147 = call "Send raw Gcode.vi"("Gcode"="M114", "VISA resource name"=w296) -> ("read buffer"=w304:string)  [unwired: 6 in, 3 out]
        n148 = Search/Split String(string=w304, search string/char (-)="Y") -> (substring before match=w306:string, match + rest of string=w305:string)  [unwired: 1 in, 1 out]
        n149 = Search/Split String(string=w305, search string/char (-)="Z") -> (substring before match=w308:string, match + rest of string=w309:string)  [unwired: 1 in, 1 out]
        n150 = String Subset(string=w306, offset (0)=2) -> (substring=w295:string)  [unwired: 1 in]
        n151 = Search/Split String(string=w309, search string/char (-)=" ") -> (substring before match=w307:string)  [unwired: 1 in, 2 out]
        n152 = String Subset(string=w308, offset (0)=2) -> (substring=w294:string)  [unwired: 1 in]
        n153 = String Subset(string=w307, offset (0)=2) -> (substring=w293:string)  [unwired: 1 in]
      }
      event "Z-": Value Change {
        (unwired) 5
        n154 = event-data() -> ()  [unwired: 1 in, 4 out]
        n155 = Format Into String(w312) -> (resulting string=w311:string)  [unwired: 3 in, 1 out]
        n156 = Concatenate Strings("G91; \nG0  Z-", w311, ";\nG90") -> (w313:string)
        n157 = call "Send raw Gcode.vi"("Gcode"=w313, "VISA resource name"=w333) -> ("VISA resource name out"=w319:refnum<visa-resource-name>)  [unwired: 6 in, 3 out]
        n158 = call "Send raw Gcode.vi"("Gcode"="M114", "VISA resource name"=w319) -> ("read buffer"=w327:string)  [unwired: 6 in, 3 out]
        n159 = Search/Split String(string=w327, search string/char (-)="Y") -> (substring before match=w329:string, match + rest of string=w328:string)  [unwired: 1 in, 1 out]
        n160 = Search/Split String(string=w328, search string/char (-)="Z") -> (substring before match=w331:string, match + rest of string=w332:string)  [unwired: 1 in, 1 out]
        n161 = String Subset(string=w329, offset (0)=2) -> (substring=w318:string)  [unwired: 1 in]
        n162 = Search/Split String(string=w332, search string/char (-)=" ") -> (substring before match=w330:string)  [unwired: 1 in, 2 out]
        n163 = String Subset(string=w331, offset (0)=2) -> (substring=w317:string)  [unwired: 1 in]
        n164 = String Subset(string=w330, offset (0)=2) -> (substring=w316:string)  [unwired: 1 in]
      }
      event "Run Scan": Mouse Down {
        w344 = ","
        # "Creates an array\nof size Nx9, where \nN is the number of\npoints that will be \nvisited during scan"
        n165 = event-data() -> ()  [unwired: 1 in, 8 out]
        n166 = Open/Create/Replace File(file path (use dialog)="Data Save Location", operation (0:open)=T1."open", access (0:read/write)=enum16{"read/write", "read-only", "write-only"}."write-only") -> (refnum out=w339:refnum<file>, error out=w337:errorcluster)  [unwired: 3 in, 1 out]
        n167 = call-poly <vilib>:"Read Delimited Spreadsheet.vi"("file path (dialog if empty)"=w346, "delimiter (\\t)"=w344) -> ("all rows"=w352:dbl[][])  [unwired: 8 in, 5 out]
        n168 = Write to Text File(file (use dialog)=w339, text="X     Y     Z     Bx     By     Bz     sigX     sigY     sigZ\n", error in=w337) -> (refnum out=w338:refnum<file>, error out=w336:errorcluster)  [unwired: 1 in, 1 out]
        n169 = Array Size(array=w352) -> (size(s)=w349:i32[])
        n170 = Index Array(array=w349, index=0) -> (element=w347:i32)
        n171 = for {
          N: w347 -> [_]
          tunnel: w352 -> [w364]
          tunnel: w351 -> [w366]
          tunnel: w348 -> [w362]
          tunnel: w345 -> [_]
          tunnel: w344 -> [_]
          tunnel: w338 -> [w357]
          tunnel: w336 -> [w355]
          shift-right: [w354] -> w341
          shift-left: _ -> [_]
          shift-right: [w353] -> w340
          shift-left: _ -> [_]
          i -> [w360]
          stop <- "Exit Scan\nClose" stop-if-true
          # "Reads into Labview the path array"
          n172 = call "gCode Generator (SubVI).vi"("row number"=w360, "Array"=w364) -> ("Position Out"=w359:string, "String"=w363:string)  [unwired: 13 in, 3 out]
          n173 = call "Send raw Gcode.vi"("Gcode"=w363, "VISA resource name"=w366) -> ("VISA resource name out"=w365:refnum<visa-resource-name>)  [unwired: 6 in, 3 out]
          n174 = flat-sequence {
            tunnel: w365 -> [w367]
            tunnel: w362 -> [w374]
            tunnel: [w372] -> w358
            tunnel: w360 -> [_]
            tunnel: w359 -> [w378]
            tunnel: w358 -> [w375]
            tunnel: [w379] -> w356
            tunnel: w357 -> [w384]
            tunnel: w356 -> [w383]
            tunnel: w355 -> [w382]
            tunnel: [w381] -> w354
            tunnel: [w380] -> w353
            frame #0 {
              n175 = while {
                tunnel: w367 -> [w370]
                stop <- w368 stop-if-true
                # "G4 P0 waits \nfor previous \ncommands to \nfinish before\nsending ok"
                # "See in testing if this\nworks. Goal is to stop \nloop once ok is read back"
                n176 = call "Send raw Gcode.vi"("Gcode"="G4 P0", "VISA resource name"=w370) -> ("command OK"=w368:bool)  [unwired: 6 in, 3 out]
              }
            }
            frame #1 {
              # "Pause to make sure \nprinter is fully stopped"
              n177 = Wait (ms)(milliseconds to wait=50) -> ()  [unwired: 1 out]
            }
            frame #2 {
              # "Expand to show more settings. Kept as constant as this works for most ports"
              # "Reads sensor"
              n178 = call "sensorReader3.0.vi"("VISA Refnum in"=w374, "Serial Settings"=T2 {"baud rate"=9600, "data bits"=8, "parity"=enum."None", "stop bits"=10, "flow control"=0}) -> ("Text Out"=w372:string)  [unwired: 13 in]
            }
            frame #3 {
              # "Inputs sensor reader\nsubVI into preallocated \narray"
              n179 = Concatenate Strings(w378, " " ("string"), w375, "\n") -> (w379:string)
            }
            frame #4 {
              n180 = Write to Text File(file (use dialog)=w384, text=w383, error in=w382) -> (refnum out=w381:refnum<file>, error out=w380:errorcluster)  [unwired: 1 in, 1 out]
            }
          }
        }
        n181 = Close File(refnum=w341, error in=w340) -> ()  [unwired: 2 out]
      }
      event "Plot Path Button": Mouse Down {
        w387 = 1
        # "Splits array into X vector"
        # "Reads Path Length"
        n182 = event-data() -> ()  [unwired: 1 in, 8 out]
        n183 = call-poly <vilib>:"Read Delimited Spreadsheet.vi"("file path (dialog if empty)"=w385, "delimiter (\\t)"=",") -> ("all rows"=w390:dbl[][])  [unwired: 8 in, 5 out]
        n184 = Array Size(array=w390) -> (size(s)=w396:i32[])
        n185 = Index Array(array=w396, index=0) -> (element=w389:i32)
        n186 = Array Subset(array=w390, index (row)=w387, length (row)=w389, index (col)=0, length (col)=w387) -> (w392:dbl[][])
        n187 = Array Subset(array=w390, index (row)=w387, length (row)=w389, index (col)=w387, length (col)=w387) -> (w391:dbl[][])
        n188 = Array Subset(array=w390, index (row)=w387, length (row)=w389, index (col)=2, length (col)=w387) -> (w397:dbl[][])
        n189 = call-poly <vilib>:"Plot Helper.vi"("z matrix"=w397, "y matrix"=w391, "x matrix"=w392) -> ("3D Plot lvclass Array out"=→"MAPPING PATH VISUALIZER (mm)":refnum<class "3D Plot Datatype.lvclass">[])  [unwired: 3 in, 5 out]
      }
      event "Close Probe\nClose 2": Value Change {
        n190 = event-data() -> ()  [unwired: 1 in, 6 out]
        n191 = VISA Close(VISA resource name=w398) -> ()  [unwired: 1 in, 1 out]
      }
    }
    "Z" <- w12
    "Y" <- w13
    "X" <- w14
  }
